vi "Interface_Asset_Map Control.vi"(8 "error in (no error)":errorcluster, 11 "Grid_Virtual in":refnum<class "Grid_Virtual.lvclass">) -> (0 "error out":errorcluster, 3 "Grid_Virtual out":refnum<class "Grid_Virtual.lvclass">)   [LabVIEW 2015, in "Grid_Virtual.lvclass"]
uses:
  Grid_Virtual.lvclass
  Grid.lvclass
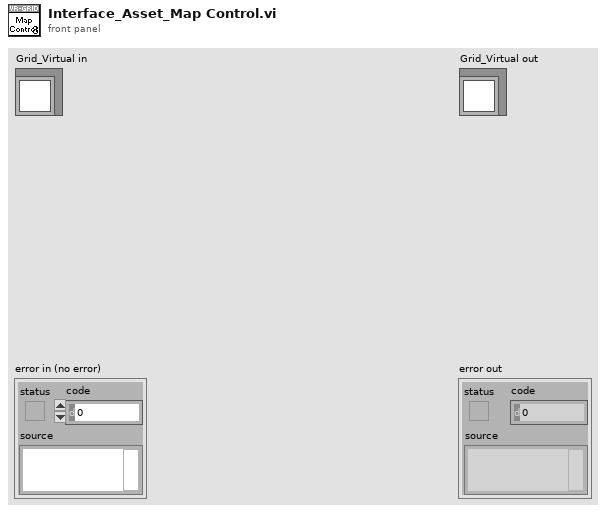
[diagram p1: front panel]
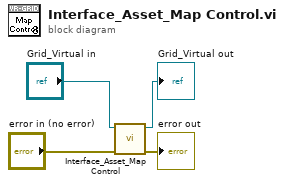
[diagram p0: block diagram]
diagram:
  n1 = call-parent "Interface_Asset_Map Control.vi"("error in (no error)"="error in (no error)", "Grid in"="Grid_Virtual in") -> ("error out"=→"error out":errorcluster, "Grid out"=→"Grid_Virtual out":refnum<class "Grid_Virtual.lvclass">)  [unwired: 8 in]
